vi "setup_lc_jd.vi"(0 "zc_luodi_num":string, 1 "jddanwei":string, 2 "jdren":string, 3 "jdlxfs":string, 4 "jddidian":string, 5 "id":string, 6 "zhriqi":string, 9 "yw":string, 14 "shuoming":string) -> (8 "error":errorcluster caption="error out 2")   [LabVIEW 2017, in "Lib_code.lvlib"]
uses:
  Lib_code.lvlib
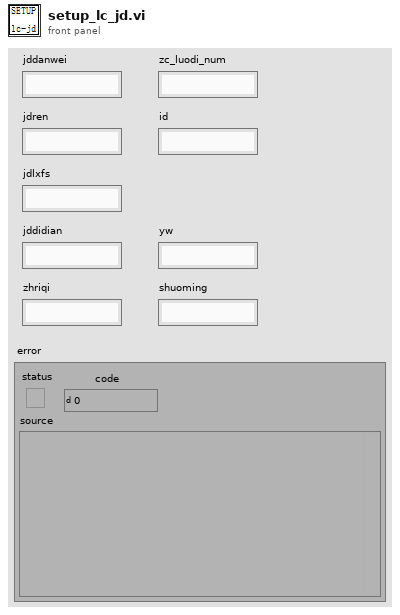
[diagram p1: front panel]
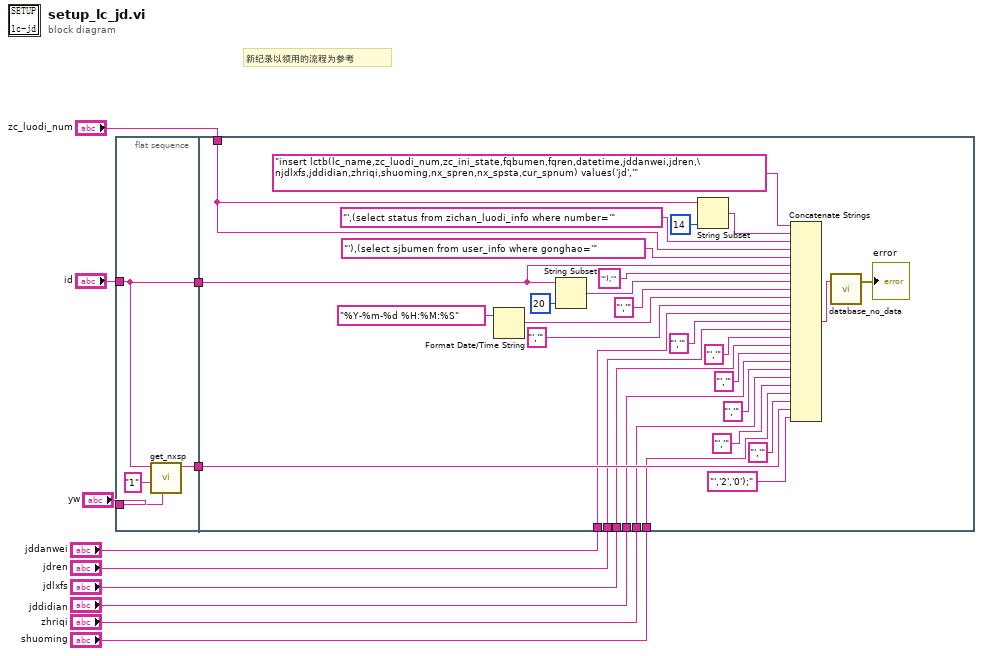
[diagram p0: block diagram]
diagram:
  # "新纪录以领用的流程为参考"
  n1 = flat-sequence {
    tunnel: "id" -> [w14]
    tunnel: [w14] -> w10
    tunnel: [w15] -> w9
    tunnel: "yw" -> [w13]
    tunnel: w10 -> [w34]
    tunnel: w9 -> [w33]
    tunnel: "zc_luodi_num" -> [w30]
    tunnel: "shuoming" -> [w25]
    tunnel: "zhriqi" -> [w23]
    tunnel: "jddidian" -> [w22]
    tunnel: "jdlxfs" -> [w21]
    tunnel: "jdren" -> [w19]
    tunnel: "jddanwei" -> [w16]
    frame #0 {
      n2 = call "get_nxsp.vi"("yw"=w13, "Cur_state"="1", "fqren"=w14) -> ("sp_gonghao"=w15:string)  [unwired: 6 in, 2 out]
    }
    frame #1 {
      n3 = Format Date/Time String(time format string (%c)="%Y-%m-%d %H:%M:%S" ("时间格式字符串(%c)")) -> (date/time string=w35:string)  [unwired: 2 in]
      n4 = String Subset(string=w34, length (rest)=20 ("长度（剩余）")) -> (substring=w37:string)  [unwired: 1 in]
      n5 = String Subset(string=w30, length (rest)=14 ("长度（剩余）")) -> (substring=w43:string)  [unwired: 1 in]
      n6 = Concatenate Strings("insert lctb(lc_name,zc_luodi_num,zc_ini_state,fqbumen,fqren,datetime,jddanwei,jdren,\njdlxfs,jddidian,zhriqi,shuoming,nx_spren,nx_spsta,cur_spnum) values('jd','" ("格式字符串"), w43, "',(select status from zichan_luodi_info where number='" ("字符串"), w30, "'),(select sjbumen from user_info where gonghao='" ("字符串"), w34, "'),'" ("字符串"), w37, "','" ("字符串"), w35, "','" ("字符串"), w16, "','" ("字符串"), w19, "','" ("字符串"), w21, "','" ("字符串"), w22, "','" ("字符串"), w23, "','" ("字符串"), w25, "','" ("字符串"), w33, "','2','0');" ("字符串")) -> (w28:string)
      n7 = call "database_no_data.vi"("input"=w28) -> ("error"=→"error":errorcluster)  [unwired: 2 in]
    }
  }
